vi "GetHistogramResultValue.vi"(8 "error in (no error)":errorcluster, 9 "data":T1, 11 "Analysis_Histogram_Parameter":T2={"Interval Range"={"Minimum"=0.0, "Maximum"=0.0}, "ROI Out"={"Global Rectangle"=[], "Contours"=[]}, "Number of Classes"=256} {"Interval Range"."Maximum" format="%.2f"; "Interval Range"."Minimum" format="%.2f"}) -> (0 "error out":errorcluster, 3 "ResultValues":string[](array[string]))   [LabVIEW 2019]
uses:
  Controls/Histogram/Analysis_Histogram_Parameter.ctl
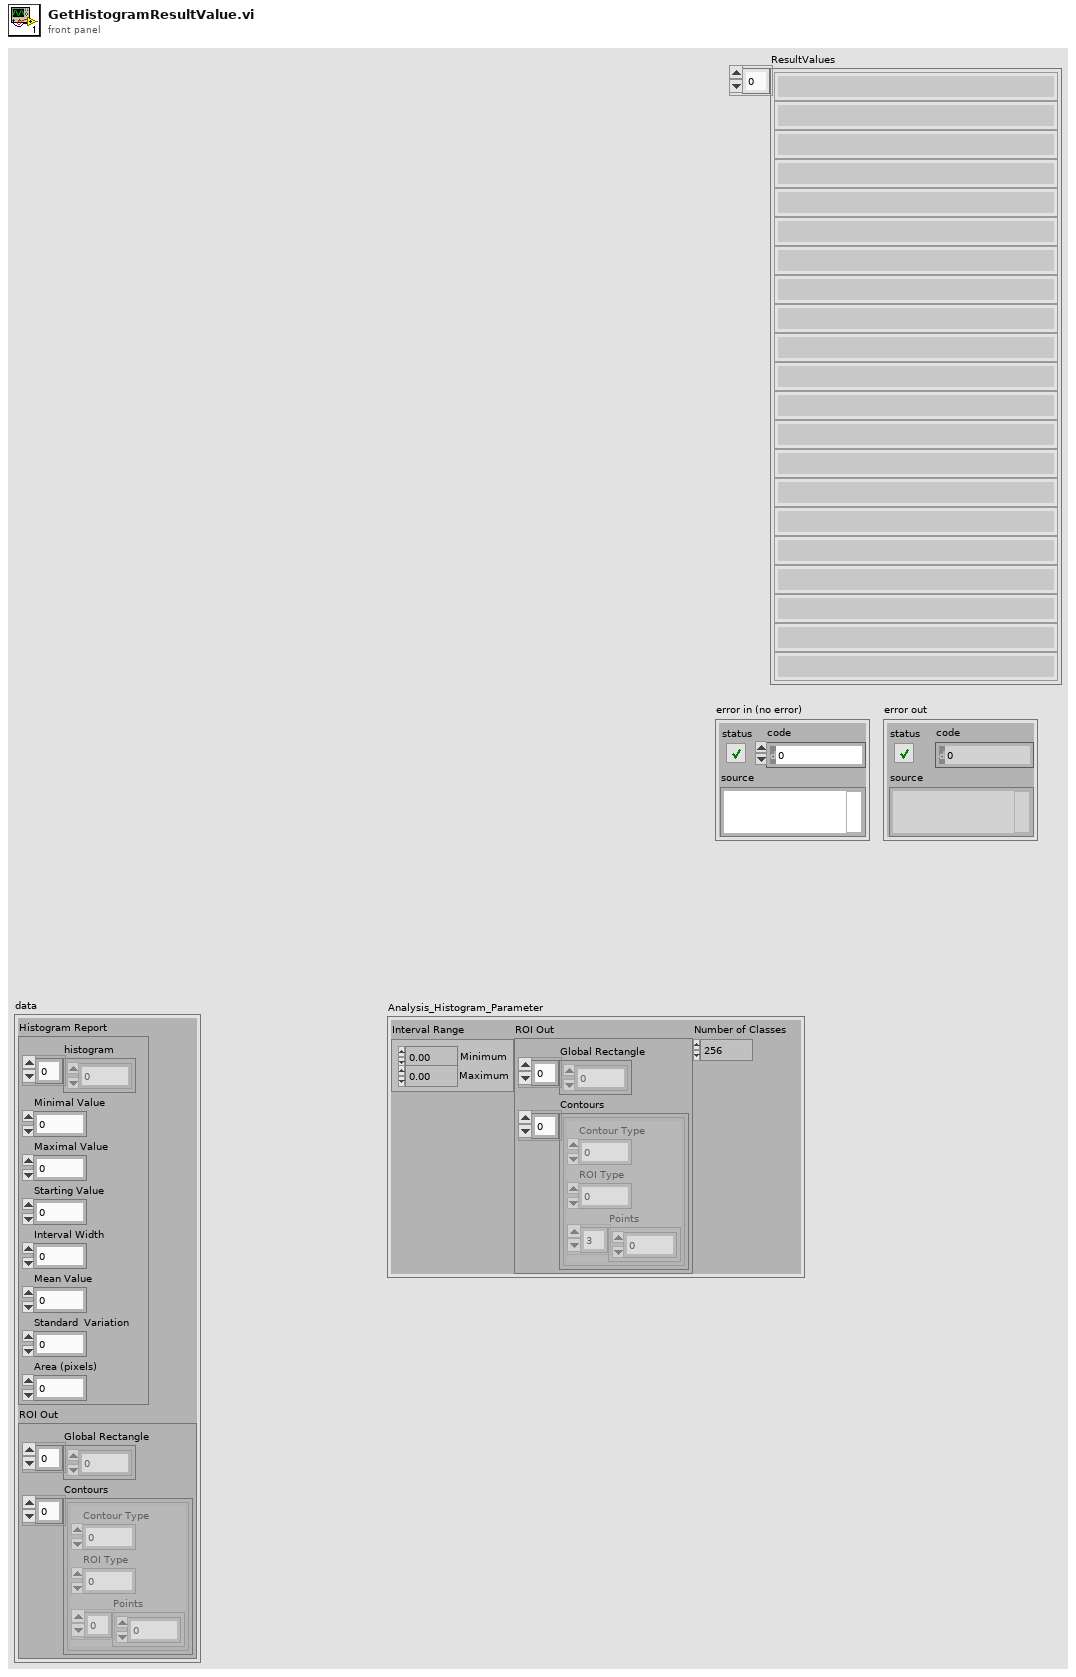
[diagram p1: front panel]
types:
  T1 = cluster{"Histogram Report":cluster{"histogram":u32[], "Minimal Value":sgl, "Maximal Value":sgl, "Starting Value":sgl, "Interval Width":sgl, "Mean Value":sgl, "Standard  Variation":sgl, "Area (pixels)":i32}, "ROI Out":cluster{"Global Rectangle":i32[], "Contours":cluster{"Contour Type":u32, "ROI Type":u32, "Points":i32[]}[]}}
  T2 = typedef "Analysis_Histogram_Parameter.ctl" = cluster{"Interval Range":cluster{"Minimum":sgl, "Maximum":sgl}, "ROI Out":cluster{"Global Rectangle":i32[], "Contours":cluster{"Contour Type":u32, "ROI Type":u32, "Points":i32[]}[]}, "Number of Classes":i32}
  T3 = cluster{"histogram":u32[], "Minimal Value":sgl, "Maximal Value":sgl, "Starting Value":sgl, "Interval Width":sgl, "Mean Value":sgl, "Standard  Variation":sgl, "Area (pixels)":i32}
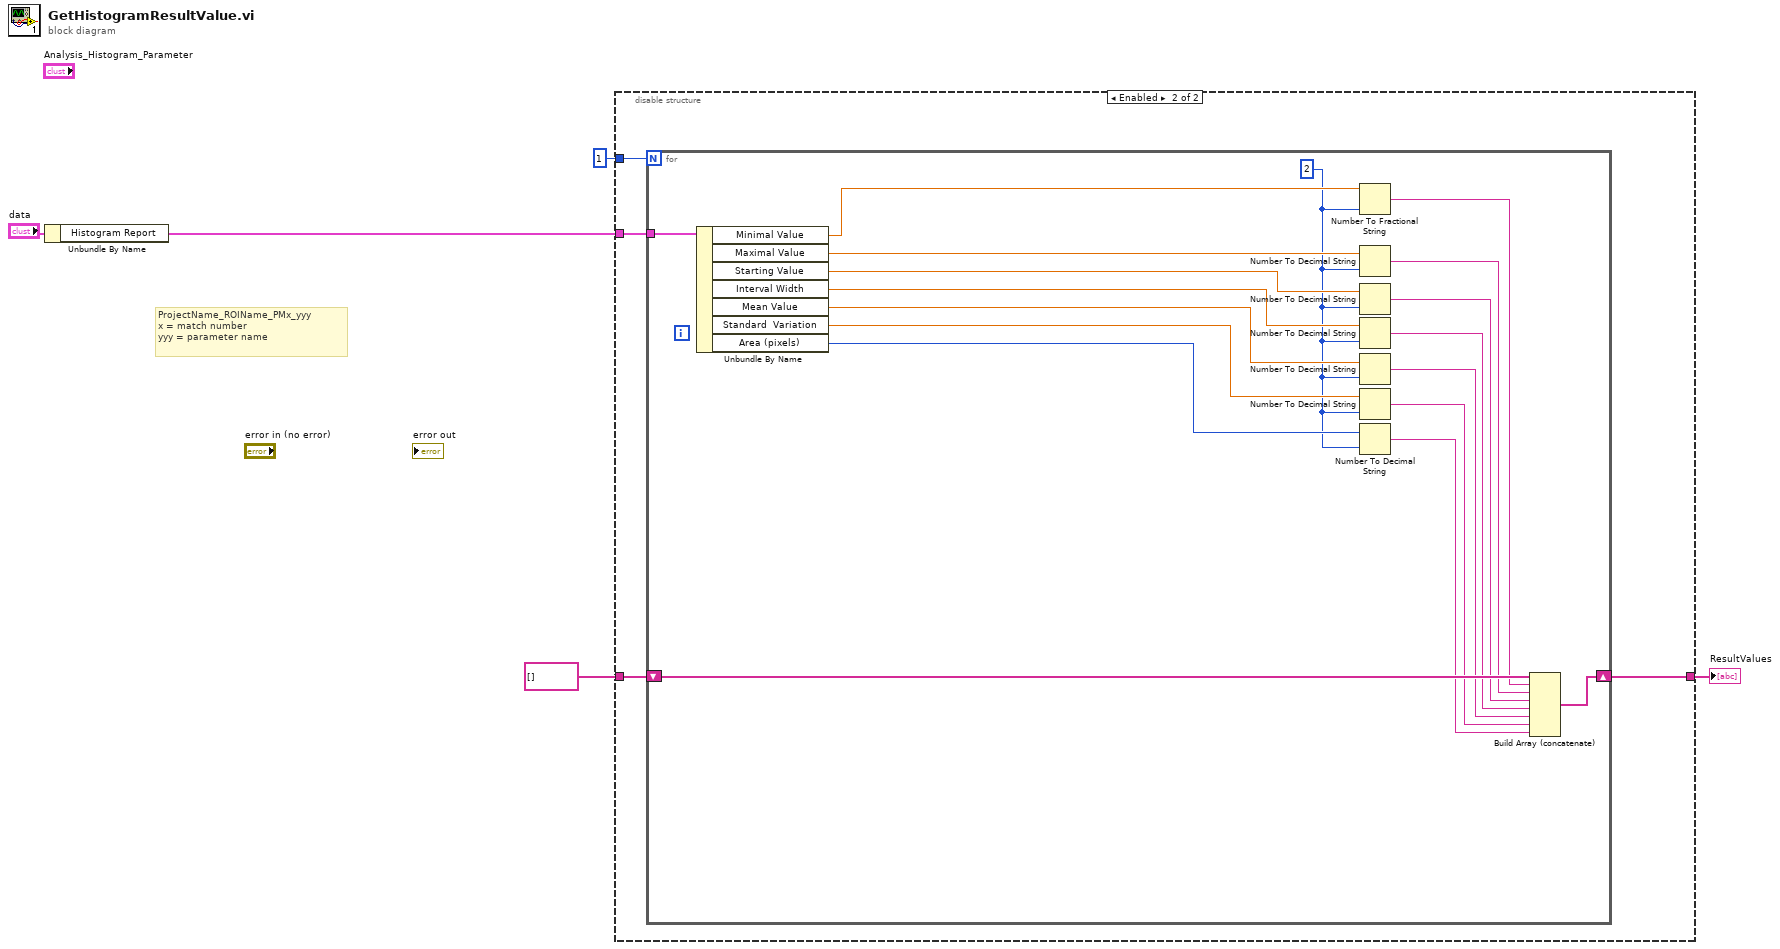
[diagram p0: block diagram]
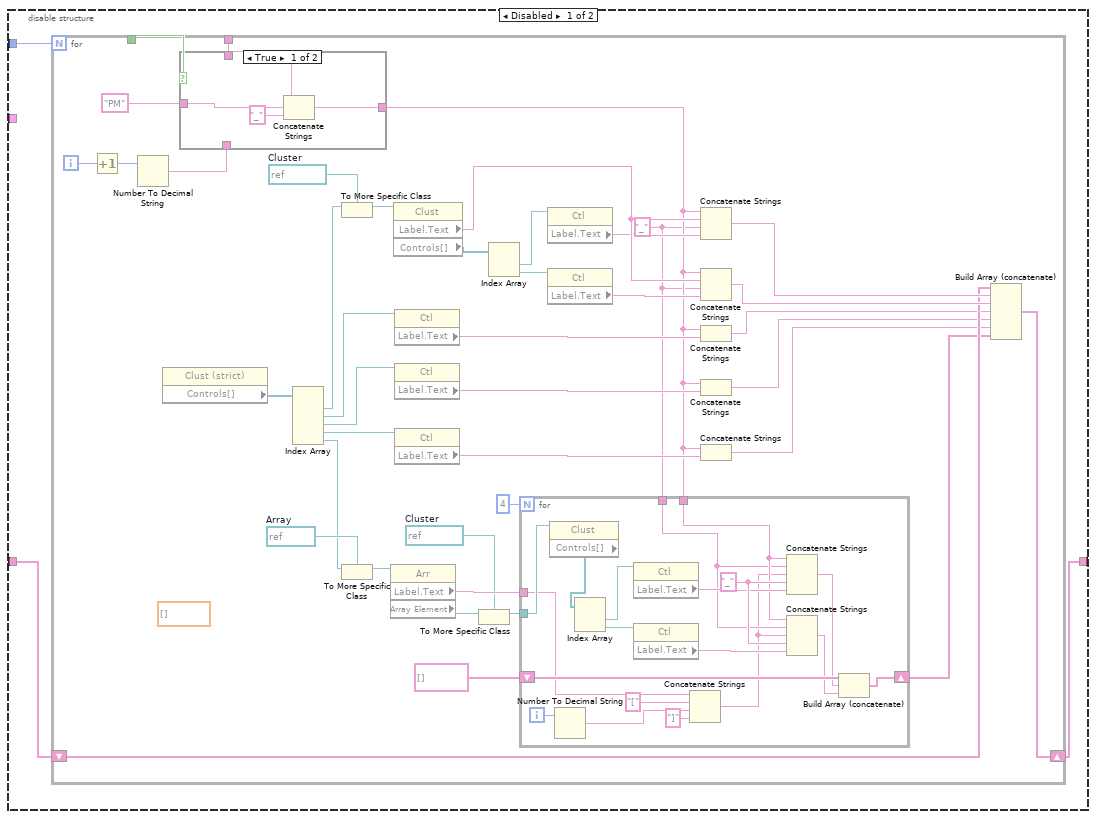
[diagram p2: hidden frame]
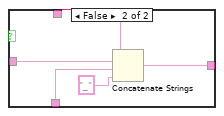
[diagram p3: hidden frame]
diagram:
  # "ProjectName_ROIName_PMx_yyy\nx = match number\nyyy = parameter name"
  n1 = Unbundle By Name("data") -> ("Histogram Report"=w1:T3)
  n2 = disable-structure shown="Enabled" {
    disable-tunnel: 1 ("Number of Matches Requested") -> [w9 w83]
    disable-tunnel: string[] [] -> [w8 w82]
    disable-tunnel: [w7 w81] -> w4
    disable-tunnel: w1 -> [_ w80]
    frame Disabled {
      n3 = for {
        N: w9 -> [_]
        tunnel: _ -> [w31]
        shift-right: [w33] -> w7
        shift-left: w8 -> [w34]
        tunnel: [w32] -> w6
        i -> [w37]
        w16 = refnum<vi> refnum  # Cluster
        (unwired) dbl[] []
        w21 = refnum<vi> refnum  # Array
        w12 = "_" ("string")
        w47 = refnum<vi> refnum  # Cluster
        n4 = Increment(x=w37) -> (x+1=w36:i32)
        n5 = Number To Decimal String(number=w36) -> (decimal integer string=w30:string)  [unwired: 1 in]
        n6 = property class="Clust (strict)"() -> (reference=w51:refnum<vi>, "Controls[]"=w50:refnum<vi>[])  [unwired: 1 in, 2 out]
        n7 = case shown="True" w32 {
          tunnel: w31 -> [w74 w79]
          tunnel: w30 -> [_ w76]
          tunnel: [w73 w78] -> w13
          tunnel: "PM" ("string") -> [w72 w75]
          frame True {
            n8 = Concatenate Strings(w74, w72, "_" ("string")) -> (w73:string)
          }
          frame False {
            n9 = Concatenate Strings(w79, w75, w76, "_" ("string")) -> (w78:string)
          }
        }
        n10 = Index Array(array=w50) -> (element #1=w49:refnum<vi>, element #2=w28:refnum<vi>, element #3=w27:refnum<vi>, element #4=w40:refnum<vi>, element #5=w20:refnum<vi>)  [unwired: 5 in]
        n11 = To More Specific Class(target class=w47, reference=w49) -> (specific class reference=w48:refnum<vi>)  [unwired: 1 in, 1 out]
        n12 = To More Specific Class(target class=w21, reference=w20) -> (specific class reference=w19:refnum<vi>)  [unwired: 1 in, 1 out]
        n13 = property class="Arr"(reference=w19) -> ("Label.Text"=w18:string, "Array Element"=w15:refnum<vi>)  [unwired: 1 in, 2 out]
        n14 = property class="Clust"(reference=w48) -> ("Label.Text"=w43:string, "Controls[]"=w46:refnum<vi>[])  [unwired: 1 in, 2 out]
        n15 = property class="Ctl"(reference=w28) -> ("Label.Text"=w26:string)  [unwired: 1 in, 2 out]
        n16 = property class="Ctl"(reference=w27) -> ("Label.Text"=w25:string)  [unwired: 1 in, 2 out]
        n17 = property class="Ctl"(reference=w40) -> ("Label.Text"=w35:string)  [unwired: 1 in, 2 out]
        n18 = To More Specific Class(target class=w16, reference=w15) -> (specific class reference=w14:refnum<vi>)  [unwired: 1 in, 1 out]
        n19 = Index Array(array=w46) -> (element #1=w45:refnum<vi>, element #2=w44:refnum<vi>)  [unwired: 2 in]
        n20 = for {
          N: 4 -> [_]
          tunnel: w18 -> [w56]
          tunnel: w14 -> [w70]
          tunnel: w13 -> [w63]
          tunnel: w12 -> [w62]
          shift-right: [w58] -> w10
          shift-left: string[] [] -> [w61]
          i -> [w57]
          w69 = "_" ("string")
          n21 = property class="Clust"(reference=w70) -> ("Controls[]"=w64:refnum<vi>[])  [unwired: 1 in, 2 out]
          n22 = Number To Decimal String(number=w57) -> (decimal integer string=w54:string)  [unwired: 1 in]
          n23 = Index Array(array=w64) -> (element #1=w65:refnum<vi>, element #2=w66:refnum<vi>)  [unwired: 2 in]
          n24 = property class="Ctl"(reference=w65) -> ("Label.Text"=w67:string)  [unwired: 1 in, 2 out]
          n25 = property class="Ctl"(reference=w66) -> ("Label.Text"=w68:string)  [unwired: 1 in, 2 out]
          n26 = Concatenate Strings(w56, "[" ("string"), w54, "]" ("string")) -> (w52:string)
          n27 = Concatenate Strings(w63, w62, w52, w69, w67) -> (w60:string)
          n28 = Concatenate Strings(w63, w62, w52, w69, w68) -> (w59:string)
          n29 = Build Array (concatenate)(w61, w60, w59) -> (w58:string[])
        }
        n30 = property class="Ctl"(reference=w45) -> ("Label.Text"=w42:string)  [unwired: 1 in, 2 out]
        n31 = property class="Ctl"(reference=w44) -> ("Label.Text"=w41:string)  [unwired: 1 in, 2 out]
        n32 = Concatenate Strings(w13, w43, w12, w42) -> (w39:string)
        n33 = Concatenate Strings(w13, w43, w12, w41) -> (w38:string)
        n34 = Concatenate Strings(w13, w26) -> (w22:string)
        n35 = Concatenate Strings(w13, w25) -> (w23:string)
        n36 = Concatenate Strings(w13, w35) -> (w24:string)
        n37 = Build Array (concatenate)(w34, w39, w38, w22, w23, w24, w10) -> (w33:string[])
      }
    }
    frame Enabled {
      n38 = for {
        N: w83 -> [_]
        shift-right: [w99] -> w81
        shift-left: w82 -> [w100]
        tunnel: w80 -> [w101]
        w84 = 2
        n39 = Unbundle By Name(w101) -> ("Minimal Value"=w98:sgl, "Maximal Value"=w90:sgl, "Starting Value"=w89:sgl, "Interval Width"=w88:sgl, "Mean Value"=w87:sgl, "Standard  Variation"=w86:sgl, "Area (pixels)"=w85:i32)
        n40 = Number To Fractional String(number=w98, precision (6)=w84) -> (F-format string=w97:string)  [unwired: 2 in]
        n41 = Number To Decimal String(number=w90, width (-)=w84) -> (decimal integer string=w96:string)
        n42 = Number To Decimal String(number=w89, width (-)=w84) -> (decimal integer string=w95:string)
        n43 = Number To Decimal String(number=w88, width (-)=w84) -> (decimal integer string=w94:string)
        n44 = Number To Decimal String(number=w87, width (-)=w84) -> (decimal integer string=w93:string)
        n45 = Number To Decimal String(number=w86, width (-)=w84) -> (decimal integer string=w92:string)
        n46 = Number To Decimal String(number=w85, width (-)=w84) -> (decimal integer string=w91:string)
        n47 = Build Array (concatenate)(w100, w97, w96, w95, w94, w93, w92, w91) -> (w99:string[])
      }
    }
  }
  "ResultValues" <- w4
